vi "Go To Connect Command .vi"() -> ()   [LabVIEW 2013, in "Receiver.lvlib" / "Receiver.lvclass"]
uses:
  Receiver.lvclass
  <vilib>/ni/Actors/State Actor/State Actor/State Actor.lvclass
  Connect Command/Connect Command.lvclass
  Receiver Commands/Receiver Commands.lvclass
panel:
  out "State out":refnum<class "State Actor.lvclass">
  out "error out":errorcluster
  in  "error in (no error)":errorcluster
  in  "Receiver.lvlib:Receiver Commands.lvlib:Receiver Commands.lvclass":refnum<class "Receiver Commands.lvclass">
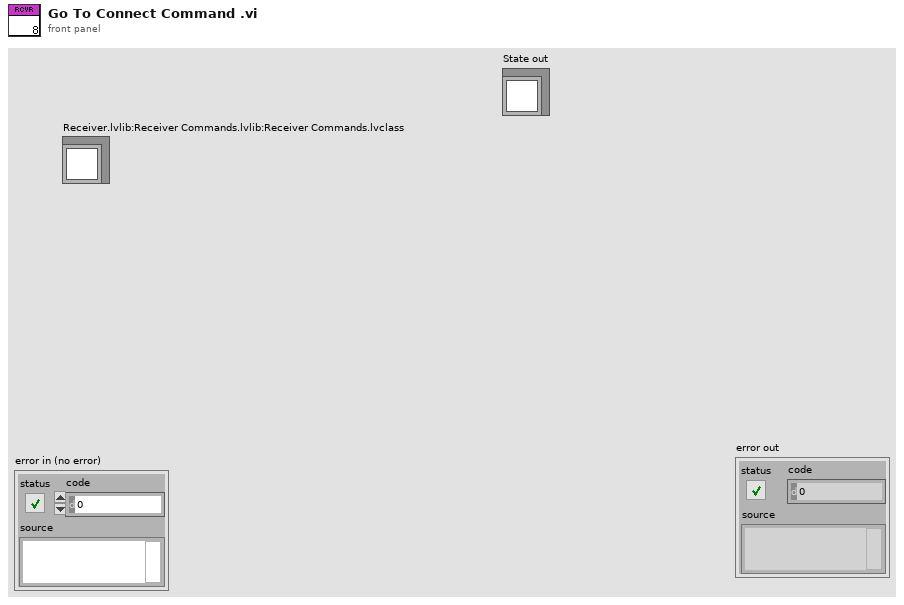
[diagram p1: front panel]
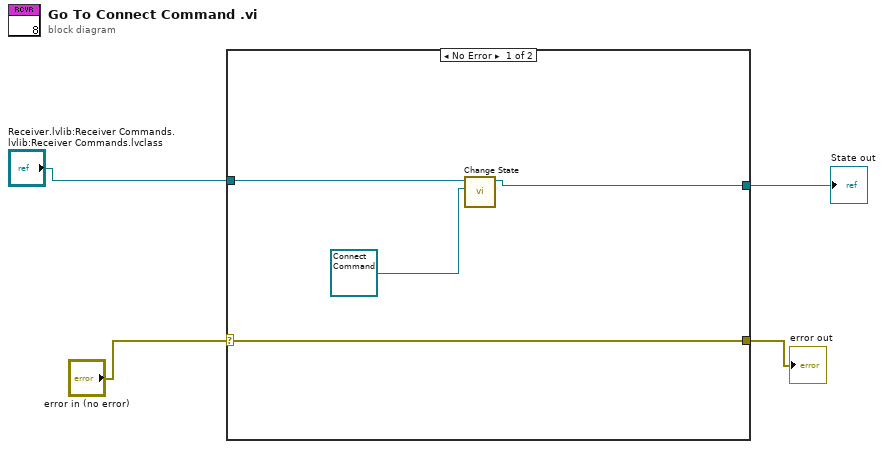
[diagram p0: block diagram]
diagram:
  n1 = case shown="No Error" "error in (no error)" {
    selector: "error in (no error)" -> [w8 w9]
    tunnel: [w8 w9] -> w3
    tunnel: "Receiver.lvlib:Receiver Commands.lvlib:Receiver Commands.lvclass" -> [w7 w10]
    tunnel: [w5 w10] -> w1
    frame No Error {
      n2 = call <vilib>:"Change State.vi"("New State in"=refnum<class "Connect Command.lvclass"> refnum ("Receiver.lvlib:Receiver Commands.lvlib:Connect Command.lvlib:Connect Command.lvclass"), "State in"=w7) -> ("State out"=w5:refnum<class "State Actor.lvclass">)  [unwired: 8 in, 1 out]
    }
    frame Error {
    }
  }
  "error out" <- w3
  "State out" <- w1
